vi "Select Indexes.vi"(8 "error in (no error)":errorcluster, 10 "Plot Indexes Array":T1[](array[typedef]), 11 "MagLabGraph in":refnum<class "XY Plot.lvclass">) -> (0 "error out":errorcluster, 3 "MagLabGraph out":refnum<class "XY Plot.lvclass">)   [LabVIEW 2015, in "XY Plot.lvclass"]
uses:
  XY Plot.lvclass
  NHMFL_Core/Libraries/Utilities/Controls/Plot Indexes.ctl
  XY Plot.lvclass/XY Plot.ctl
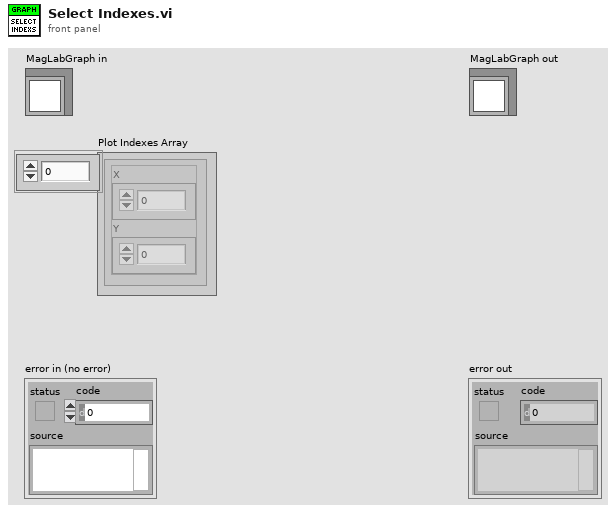
[diagram p1: front panel]
types:
  T1 = typedef "Plot Indexes.ctl" = cluster{"X":u16, "Y":u16}
  T2 = cluster{"File Path Control":path, "Group":string, "Channel":string, "Abbreviated":string}[]
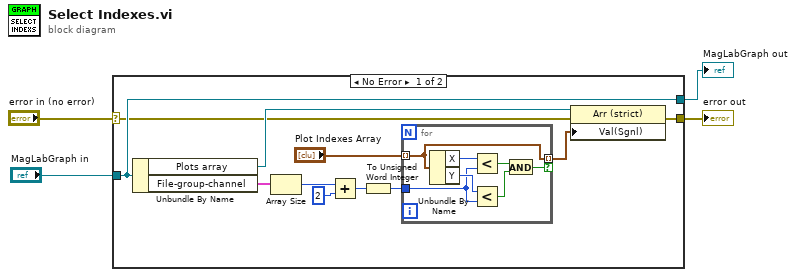
[diagram p0: block diagram]
diagram:
  n1 = case shown="No Error" "error in (no error)" {
    selector: "error in (no error)" -> [w6 w24]
    tunnel: [w5 w24] -> w3
    tunnel: [w15 w23] -> w1
    tunnel: "MagLabGraph in" -> [w15 w23]
    frame No Error {
      n2 = Unbundle By Name(w15) -> ("Plots array"=w8:refnum<vi>, "File-group-channel"=w14:T2)
      n3 = Array Size(array=w14) -> (size(s)=w13:i32)
      n4 = Add(x=w13, y=2) -> (x+y=w11:i32)
      n5 = To Unsigned Word Integer(number=w11) -> (unsigned 16bit integer=w10:u16)
      n6 = for {
        tunnel: "Plot Indexes Array" -> [w19] mode=indexing
        tunnel: w10 -> [w20]
        tunnel: [w19] -> w7 mode=indexing if=w16
        n7 = Unbundle By Name(w19) -> ("X"=w22:u16, "Y"=w21:u16)
        n8 = Less?(x=w22, y=w20) -> (x < y?=w18:bool)
        n9 = Less?(x=w21, y=w20) -> (x < y?=w17:bool)
        n10 = And(x=w18, y=w17) -> (x .and. y?=w16:bool)
      }
      n11 = property class="Arr (strict)"(reference=w8, error in=w6, "Val(Sgnl)"=w7) -> (error out=w5:errorcluster)  [unwired: 1 out]
    }
    frame Error {
    }
  }
  "error out" <- w3
  "MagLabGraph out" <- w1
